vi "GUI_TRA_TREX.vi"() -> ()   [LabVIEW 2013]
uses:
  Device Drivers/TRAServer/HomingType_TypDef.ctl
  Device Drivers/TRAServer/StatusTRA_TypDef.ctl
  Device Drivers/shared/OnOffTypeDef.ctl
  <vilib>/Utility/file.llb/Write To Spreadsheet File (string).vi
  Device Drivers/TRAServer/TRAServer.lvclass
panel:
  in  "Multicolumn Listbox 2":refnum<vi>
  in  "Main Tap 2":refnum<vi>
  out "all pos array":refnum<vi>[][](array[refnum])
  out "all status array":refnum<vi>[][](array[refnum])
  out "indecator ref array 2":refnum<vi>[](array[refnum])
  out "indecator ref array":refnum<vi>[](array[refnum])
  in  "time to wait (TCP) 2":i32=10
  in  "plot":bool=TRUE
  out "ratio(h)":bool
  out "fixsize":bool
  out "error (h)":bool
  out "Device Name (h)":string="StagingTRA1"
  in  "Main Tap":T1(tab)
  in  "stepSize":dbl=0.01
  in  "Status":T2=enum."DISABLE" caption="Status Y"
  in  "Up":bool
  in  "Down":bool
  in  "Right":bool
  in  "Left":bool
  in  "Status":T2=enum."DISABLE" caption="Status X"
  in  "Position":dbl=2.54999 caption="X"
  in  "Position":dbl=3.05 caption="Y"
  in  "Mirror":enum16{"M20", "Switch", "M22", "M23"}(ring)
  in  "device status":string
  in  "Home 3":bool=TRUE
  in  "Home 2":bool=TRUE
  out "Status.Axis 6":T2=enum."DISABLE" caption="Status X"
  out "Status.Axis 5":T2=enum."DISABLE" caption="Status X"
  out "Status.Axis 4":T2=enum."DISABLE" caption="Status X"
  out "Status.Axis 3":T2=enum."DISABLE" caption="Status X"
  out "Status.Axis 2":T2=enum."DISABLE" caption="Status X"
  out "Status.Axis 1":T2=enum."DISABLE" caption="Status X"
  out "Status.Axis 1":T2=enum."DISABLE" caption="Status X"
  out "Status.Axis 2":T2=enum."DISABLE" caption="Status X"
  out "Status.Axis 3":T2=enum."DISABLE" caption="Status X"
  out "Status.Axis 4":T2=enum."DISABLE" caption="Status X"
  out "Status.Axis 5":T2=enum."DISABLE" caption="Status X"
  out "Status.Axis 6":T2=enum."DISABLE" caption="Status X"
  out "Status.Axis 7":T2=enum."DISABLE" caption="Status X"
  out "Status.Axis 8":T2=enum."DISABLE" caption="Status X"
  out "Status.Axis 9":T2=enum."DISABLE" caption="Status X"
  out "Status.Axis 10":T2=enum."DISABLE" caption="Status X"
  out "Status.Axis 11":T2=enum."DISABLE" caption="Status X"
  out "Status.Axis 12":T2=enum."DISABLE" caption="Status X"
  in  "Home 1":bool=TRUE
  in  "Path":path
  in  "Save":bool
  in  "Multicolumn Listbox":i32(listbox)
  in  "Position.Axis 1":dbl=3.05 caption="X"
  in  "Position.Axis 2":dbl=3.05 caption="Y"
  in  "Position.Axis 4":dbl=3.05 caption="X"
  in  "Position.Axis 3":dbl=3.05 caption="Y"
  in  "Position.Axis 6":dbl=3.05 caption="X"
  in  "Position.Axis 5":dbl=3.05 caption="Y"
  in  "Position.Axis 18":dbl=3.05 caption="X"
  in  "Position.Axis 17":dbl=3.05 caption="Y"
  in  "Position.Axis 16":dbl=3.05 caption="X"
  in  "Position.Axis 15":dbl=3.05 caption="Y"
  in  "Position.Axis 14":dbl=3.05 caption="X"
  in  "Position.Axis 13":dbl=3.05 caption="Y"
  in  "Position.Axis 12":dbl=3.05 caption="X"
  in  "Position.Axis 11":dbl=3.05 caption="Y"
  in  "Position.Axis 10":dbl=3.05 caption="X"
  in  "Position.Axis 9":dbl=3.05 caption="Y"
  in  "Position.Axis 8":dbl=3.05 caption="Y"
  in  "Position.Axis 7":dbl=3.05 caption="X"
  in  "Boolean":bool
  out "local Port":u16=65435
  in  "timeout ms (slow resp)":i32=500
  in  "reset":bool
  out "image con closed":bool
  out "image \nconnection":bool
  out "image con closed 2":bool
  out "All Devices (h)":string[](array[string])=["StagingTRA1"]
  out "Remote Host":string="192.168.11.97"
  out "port or service name":u16=65434
  out "port or service name out":u16=65400
  in  "time to wait (TCP)":i32=10
  out "error out":errorcluster
  out "connections (hidden)":variant[](array[variant])=[variant(refnum<k16> refnum), variant(refnum<k16> refnum)]
  in  "time to wait (main loop)":i32=10
  out "Data String":string="Position.Axis 1,2.549990000000\r\nStatus.Axis 1,DISABLE\r\nHomingType.Axis 1,EoR- switch only\r\nDisable.Axis 1,on\r\nDisable.Axis 2,on\r\nStatus.Axis 2,DISABLE\r\nPosition.Axis 2,3.050000000000\r\n"
  in  "Local Saving Path":path
  out "Nr.":i32
  out "error (h) 2":bool
  in  "shotnumber":i32
  out "String":string="wait>>Status.Axis 1,Status.Axis 2,Status.Axis 3,Status.Axis 4,Status.Axis 5,Status.Axis 6,Position.Axis 1,Position.Axis 2,Position.Axis 3,Position.Axis 4,Position.Axis 5,Position.Axis 6,Disable.Axis 1,Disable.Axis 2,Disable.Axis 3,Disable.Axis 4,Disable.Axis 5,Disable.Axis 6,HomingType.Axis 1,HomingType.Axis 2,HomingType.Axis 3,HomingType.Axis 4,HomingType.Axis 5,HomingType.Axis 6,Home.Axis 1,Home.Axis 2,Home.Axis 3,Home.Axis 4,Home.Axis 5,Home.Axis 6,Limits.pos.Axis 1,Limits.pos.Axis 2,Limits.pos.Axis 3,Limits.pos.Axis 4,Limits.pos.Axis 5,Limits.pos.Axis 6,Limits.neg.Axis 1,Limits.neg.Axis 2,Limits.neg.Axis 3,Limits.neg.Axis 4,Limits.neg.Axis 5,Limits.neg.Axis 6,TargetPos.Axis 1,TargetPos.Axis 2,TargetPos.Axis 3,TargetPos.Axis 4,TargetPos.Axis 5,TargetPos.Axis 6,backlash.Axis 1,backlash.Axis 2,backlash.Axis 3,backlash.Axis 4,backlash.Axis 5,backlash.Axis 6"
  in  "Limits.pos":dbl=2.54999
  in  "Home":T3=enum."on"
  in  "Disable":T3=enum."on"
  in  "HomingType":T4=enum."EoR- switch only"
  in  "Disable":T3=enum."on"
  in  "HomingType":T4=enum."EoR- switch only"
  in  "Home":T3=enum."on"
  in  "Limits.pos":dbl=2.54999
  in  "Limits.neg":dbl=2.54999
  in  "Limits.neg":dbl=2.54999
  in  "Mirror 2":enum16{"M20", "Switch", "M22", "M23"}(ring)
  in  "backlash 2":dbl
  in  "backlash":dbl
  out "error message":string
  out "Data Connection out":bool=TRUE
  # "Position"
  # "Chassi 1"
  # "Chassi 2"
  # "Chassi 3"
  # "X"
  # "Y"
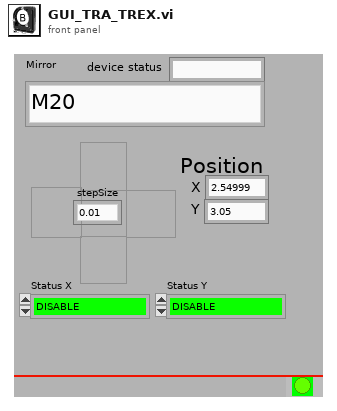
[diagram p1: front panel]
types:
  T1 = enum32{"Main", "Status", "Position", "Position 2", "Temp", "Network", "Internal", "MotorSettings"}
  T2 = typedef "TRAServer.lvclass/StatusTRA_TypDef.ctl" = enum16{"NOT REFERENCED", "CONFIGURATION", "HOMING", "MOVING", "READY", "DISABLE", "JOGGING"}
  T3 = typedef "OnOffTypeDef.ctl" = enum16{"off", "on"}
  T4 = typedef "TRAServer.lvclass/HomingType_TypDef.ctl" = enum16{"MZ switch and encoder Index", "current position as HOME", "MZ switch only", "EoR- switch and encoder Index", "EoR- switch only"}
  T5 = cluster{"Chassi Nr":i32, "X":string, "Y":string, "name":string}[]
  T6 = cluster{"Chassi Nr":i32, "X":string, "Y":string, "name":string}
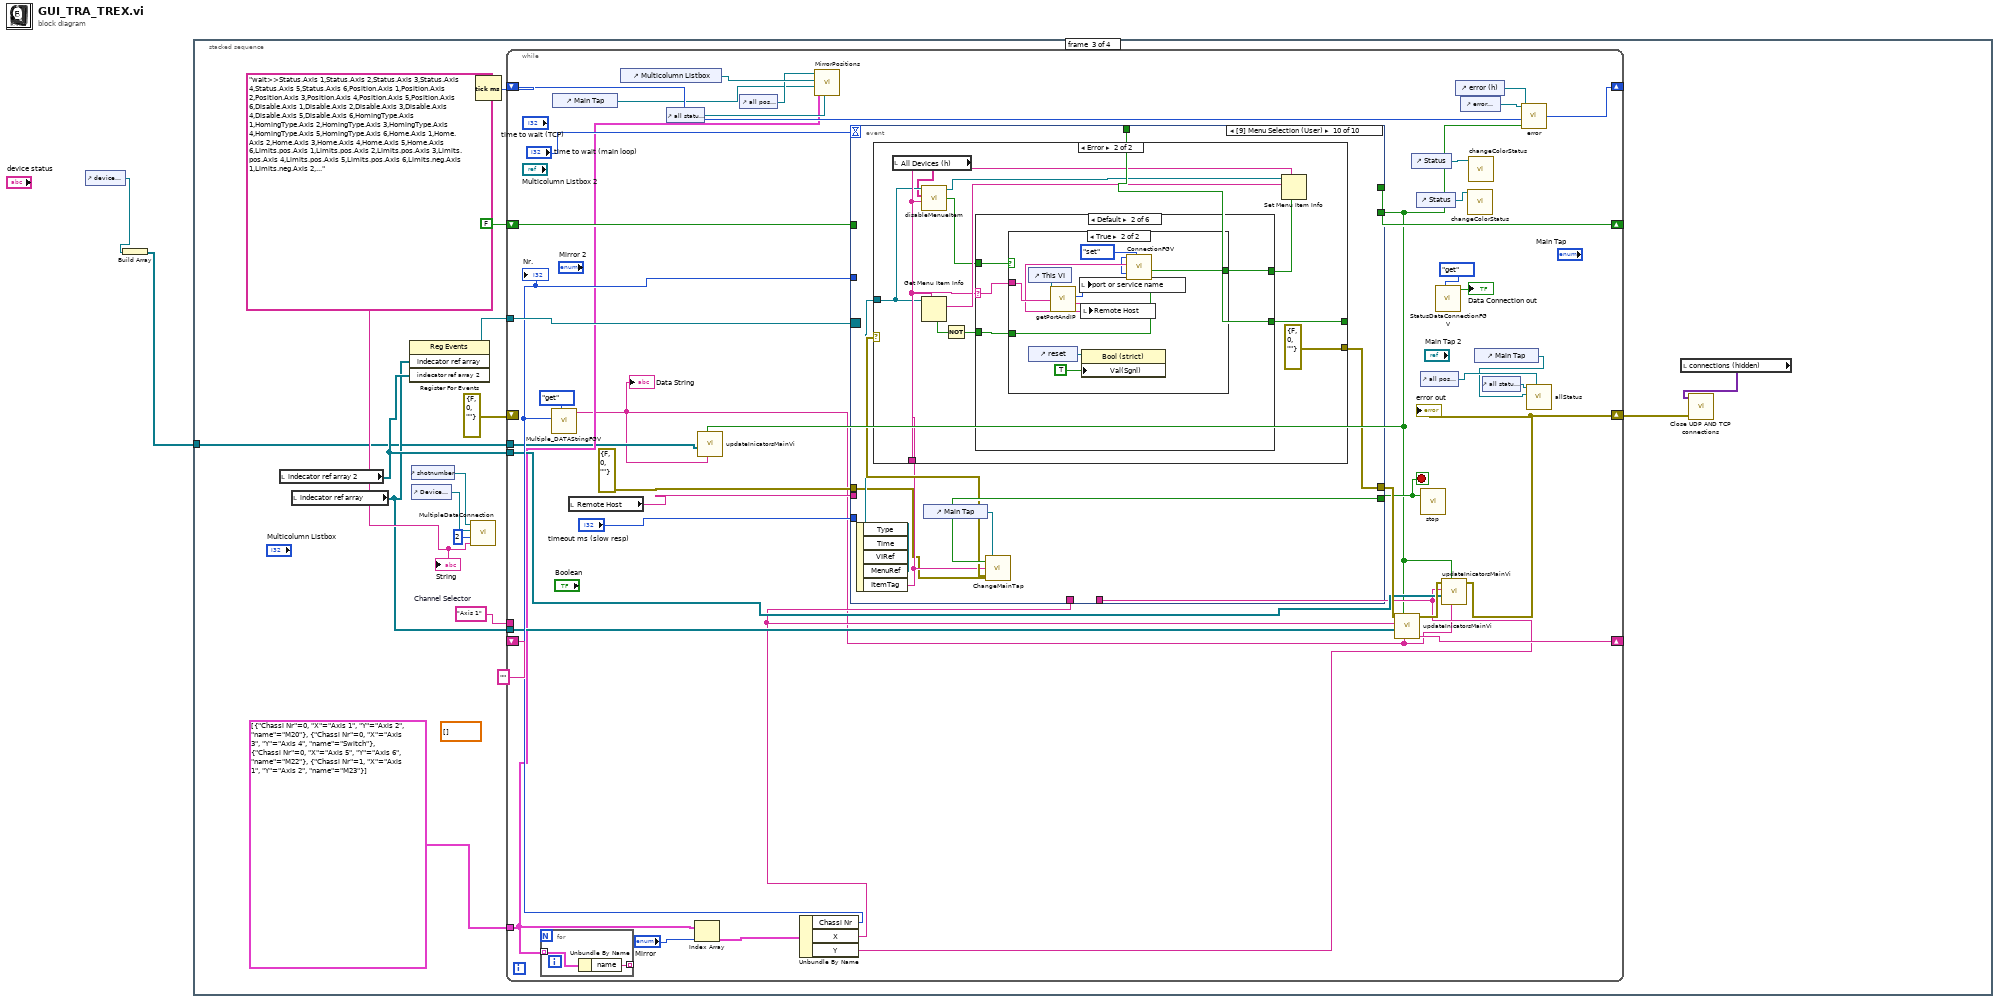
[diagram p0: block diagram]
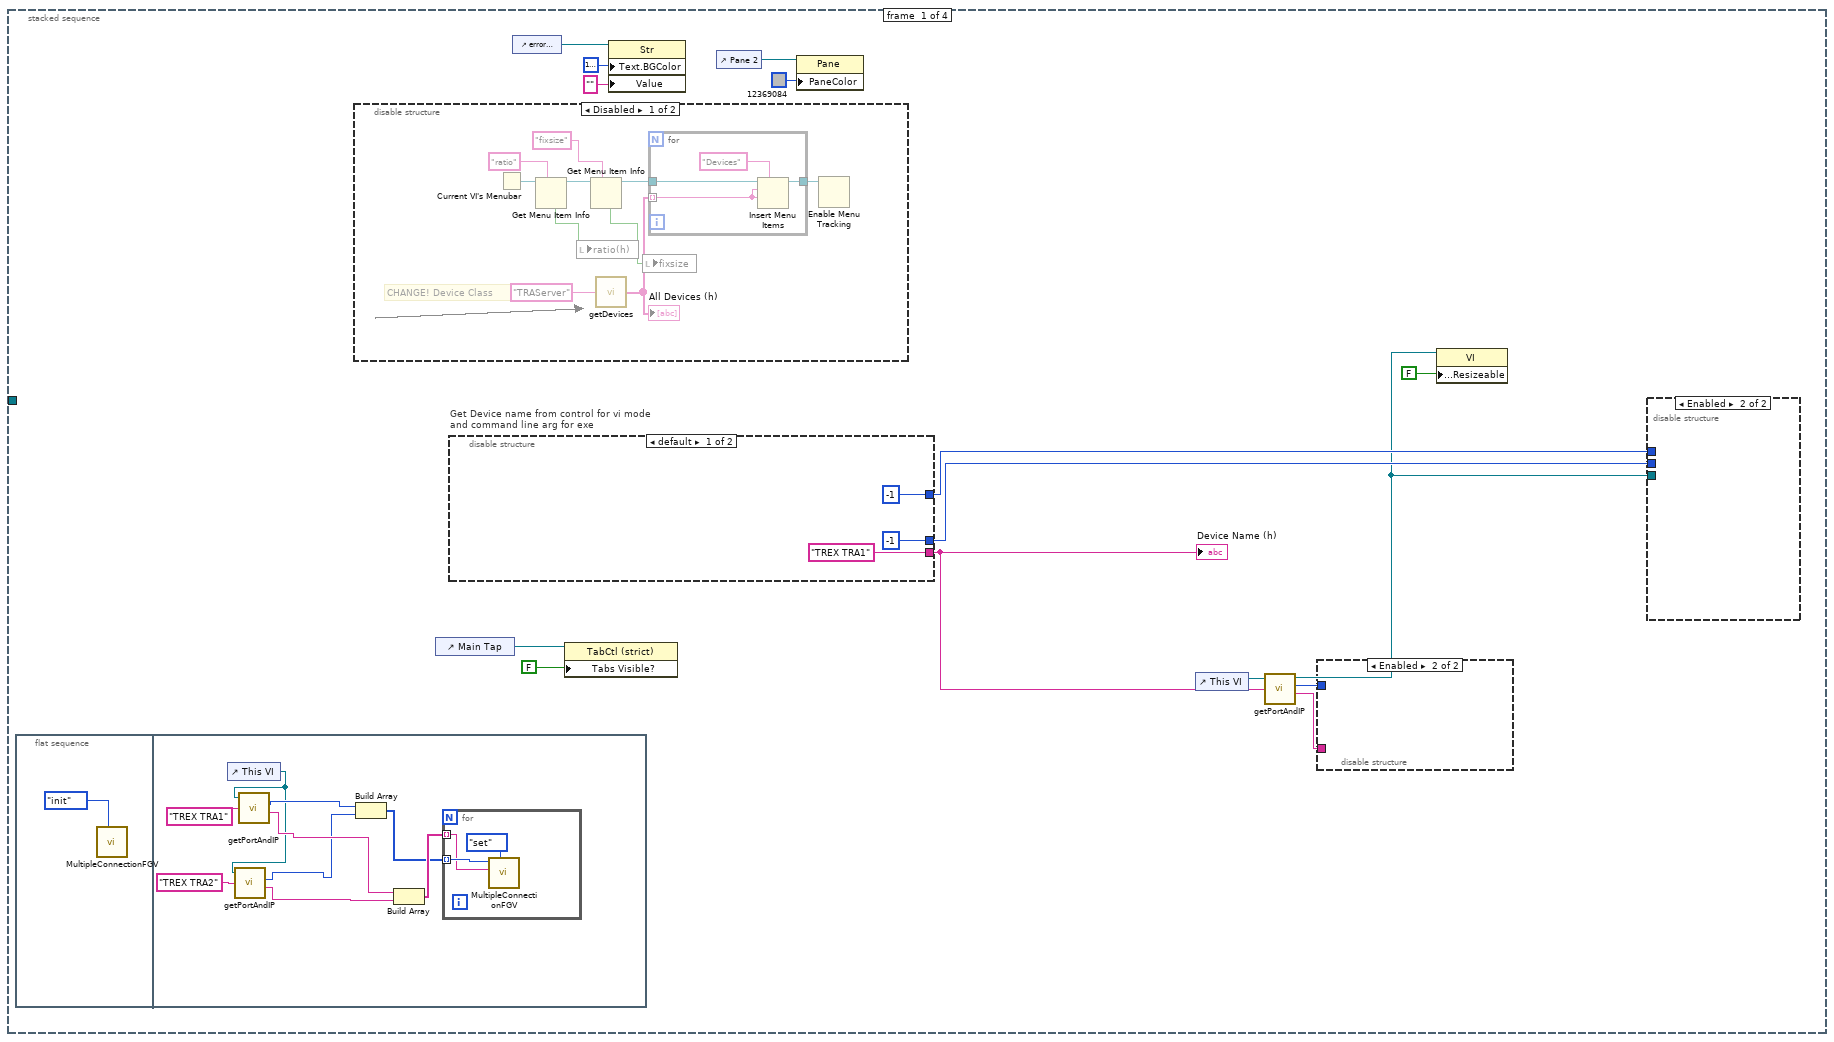
[diagram p2: hidden frame]
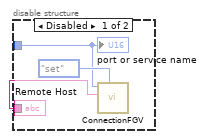
[diagram p4: hidden frame]
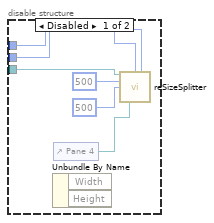
[diagram p5: hidden frame]
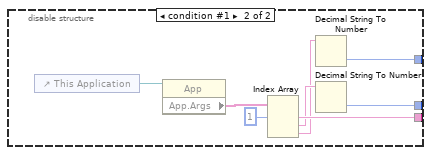
[diagram p6: hidden frame]
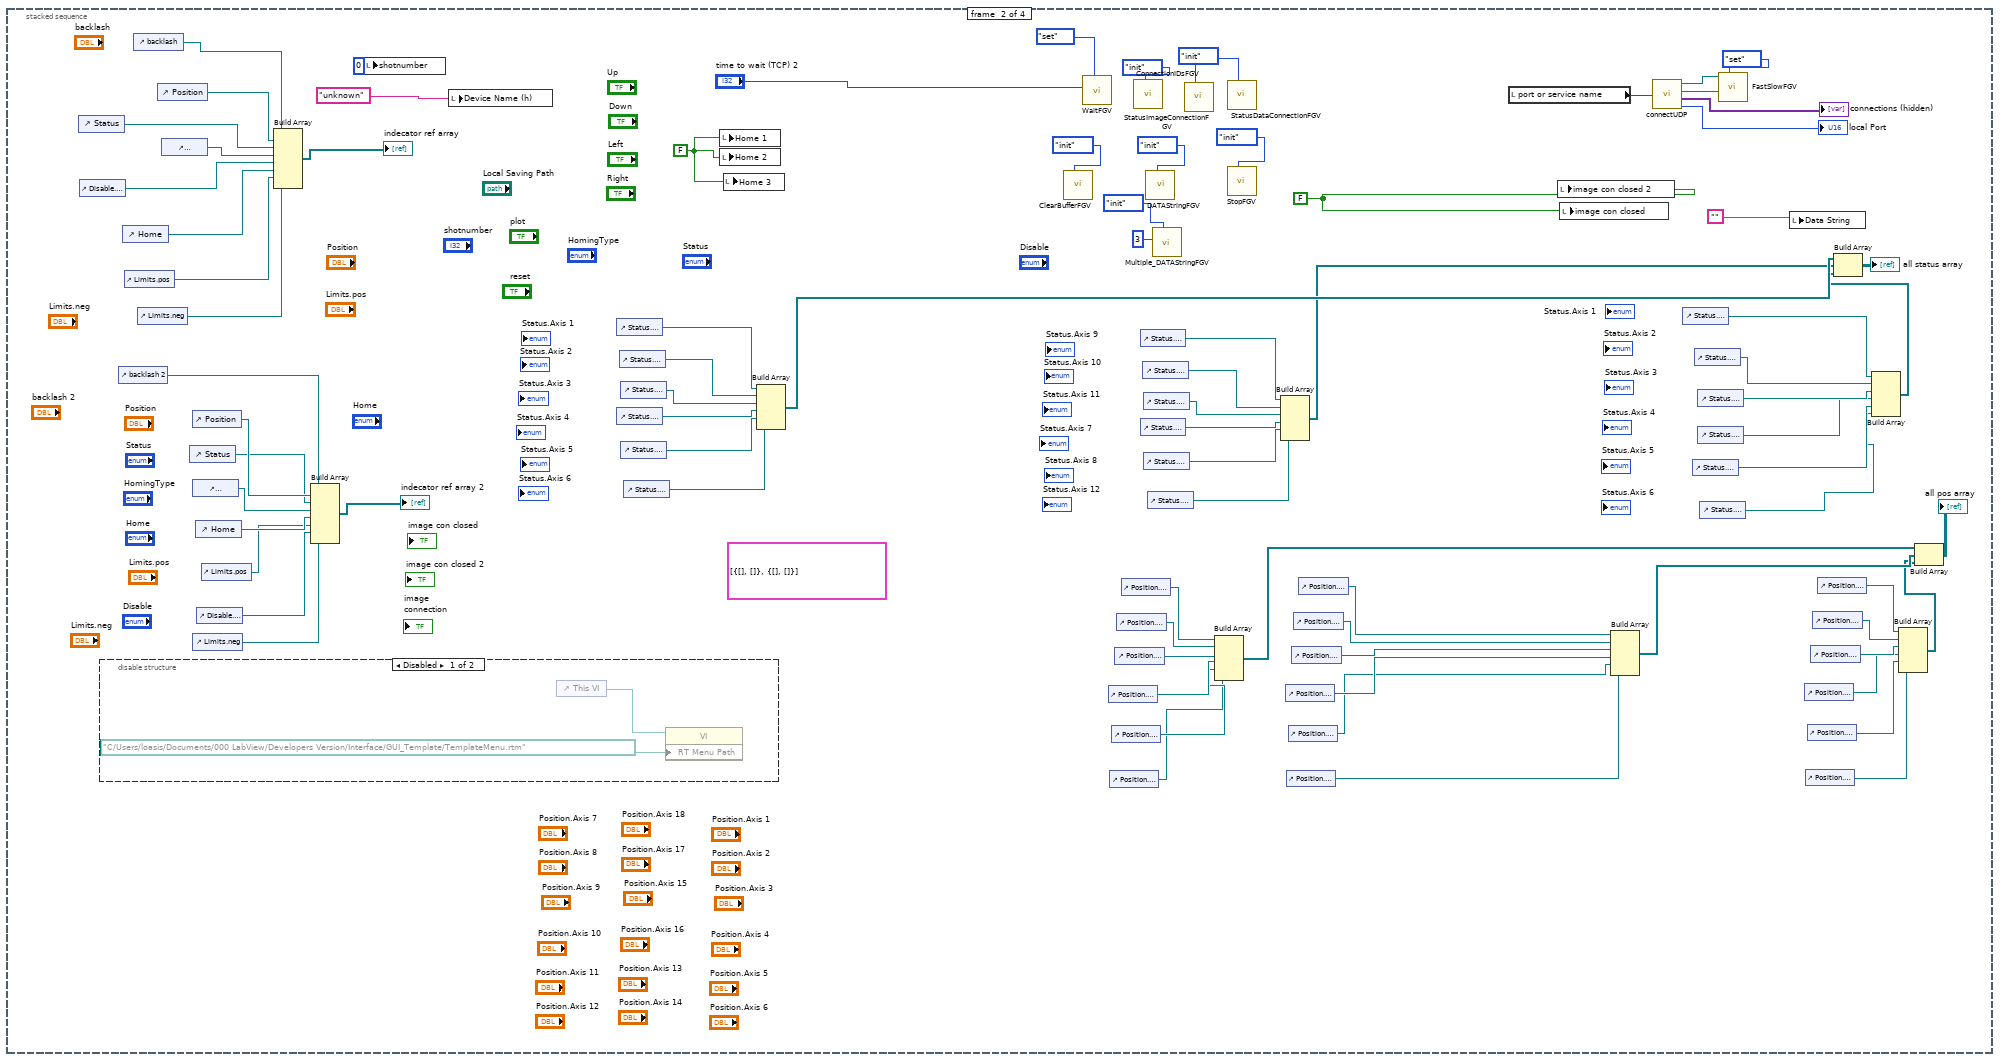
[diagram p7: hidden frame]
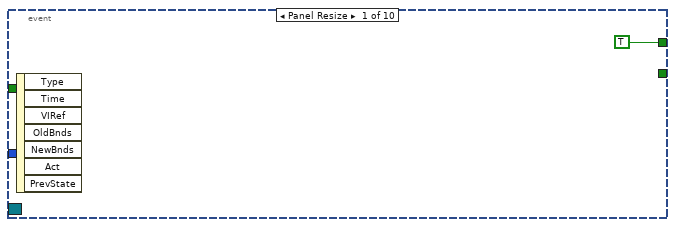
[diagram p9: hidden frame]
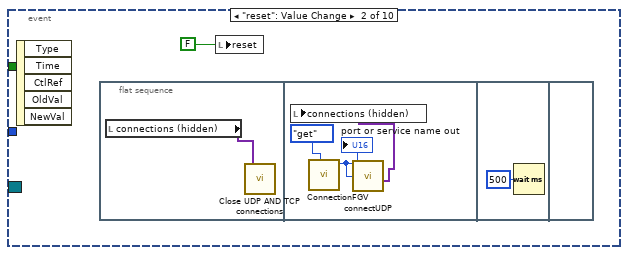
[diagram p10: hidden frame]
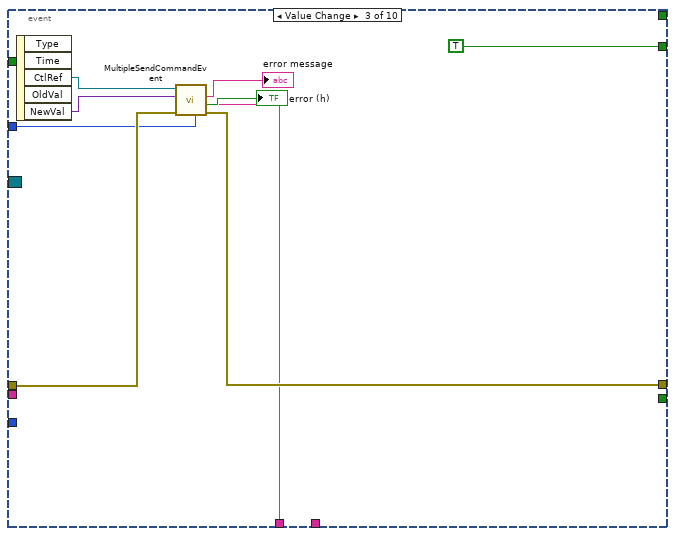
[diagram p11: hidden frame]
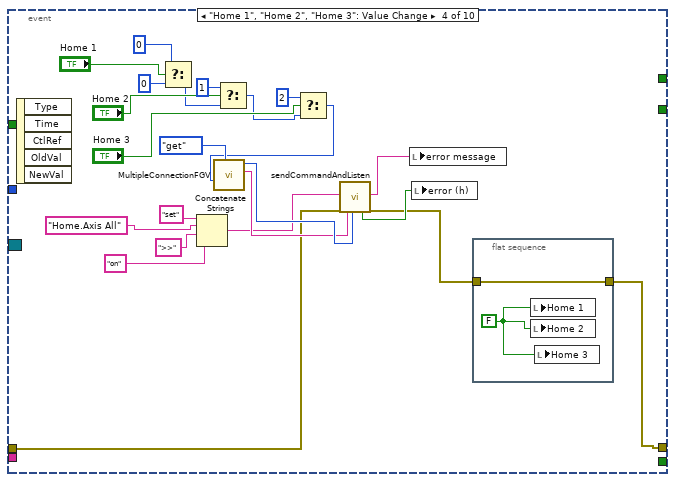
[diagram p12: hidden frame]
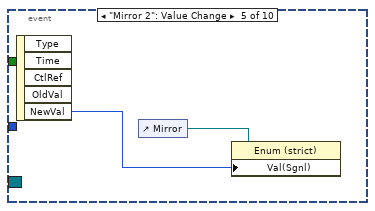
[diagram p13: hidden frame]
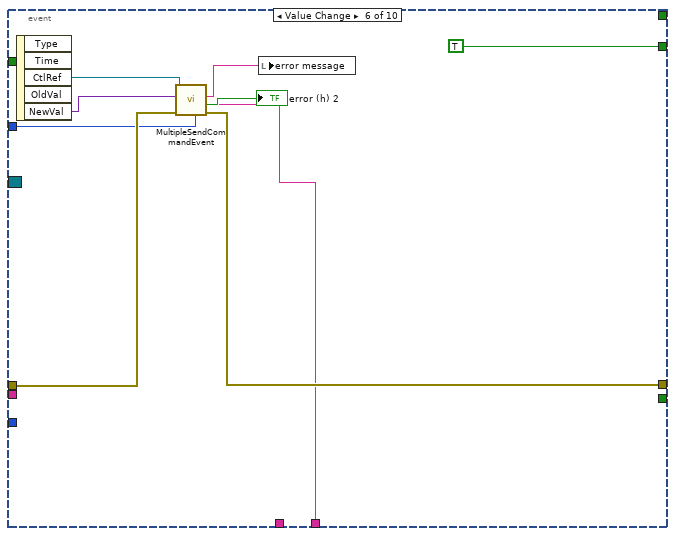
[diagram p14: hidden frame]
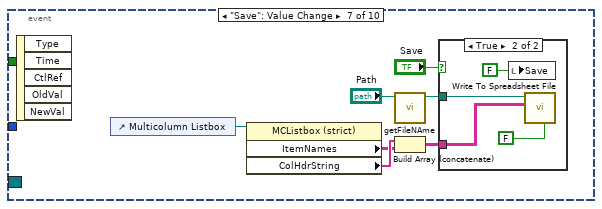
[diagram p15: hidden frame]
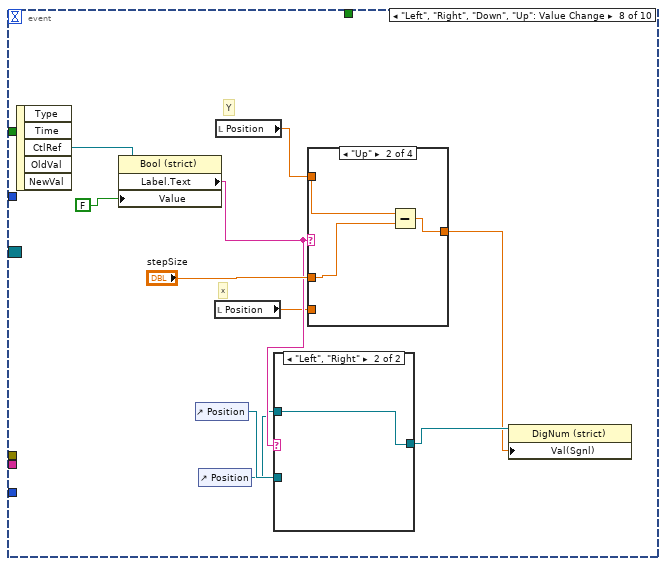
[diagram p17: hidden frame]
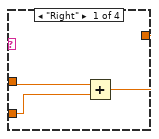
[diagram p19: hidden frame]
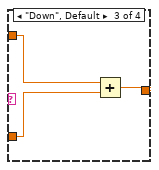
[diagram p20: hidden frame]
diagram:
  n1 = control-ref of="device status"() -> (w2:refnum<vi>)
  n2 = Build Array(w2) -> (w1:refnum<vi>[])
  n3 = stacked-sequence {
    tunnel: w1 -> [_ _ w149 _]
    frame #0 {
      n4 = flat-sequence {
        frame #0 {
          n5 = call "MultipleConnectionFGV.vi"("command"=enum16{"get", "set", "init"}."init") -> ()  [unwired: 9 in, 2 out]
        }
        frame #1 {
          n6 = control-ref of="This VI"() -> (w35:refnum<vi>)
          n7 = call "getPortAndIP.vi"("Device Name"="TREX TRA2", "This Vi"=w35) -> ("Remote Host"=w34:string, "port or service name"=w33:u16)  [unwired: 2 in, 3 out]
          n8 = call "getPortAndIP.vi"("Device Name"="TREX TRA1", "This Vi"=w35) -> ("Remote Host"=w38:string, "port or service name"=w37:u16)  [unwired: 2 in, 3 out]
          n9 = Build Array(w37, w33) -> (w40:u16[])
          n10 = Build Array(w38, w34) -> (w41:string[])
          n11 = for {
            tunnel: w40 -> [w43] mode=indexing
            tunnel: w41 -> [w42] mode=indexing
            n12 = call "MultipleConnectionFGV.vi"("command"=enum16{"get", "set", "init"}."set", "Remote Host in"=w42, "port or service name in"=w43) -> ()  [unwired: 7 in, 2 out]
          }
        }
      }
      n13 = disable-structure shown="Disabled" {
        frame Disabled {
          # "CHANGE! Device Class"
          n14 = Current VI's Menubar() -> (w26:refnum<k9>)
          n15 = Get Menu Item Info(7:"ratio" ("item tag"), 11:w26) -> (3:w24:refnum<k9>, 4:w25:bool)  [unwired: 1 in, 5 out]
          n16 = local write "ratio(h)"(w25) -> ()
          n17 = Get Menu Item Info(7:"fixsize" ("item tag"), 11:w24) -> (3:w21:refnum<k9>, 4:w22:bool)  [unwired: 1 in, 5 out]
          n18 = call "getDevices.vi"("Device Class"="TRAServer") -> ("All Devices"=w19:string[])
          "All Devices (h)" <- w19
          n19 = local write "fixsize"(w22) -> ()
          n20 = for {
            tunnel: w21 -> [w31]
            tunnel: [w30] -> w20
            tunnel: w19 -> [w28] mode=indexing
            n21 = Insert Menu Items(5:"Devices" ("menu tag"), 7:w28, 8:w28, 9:w31) -> (3:w30:refnum<k9>)  [unwired: 2 in, 2 out]
          }
          n22 = Enable Menu Tracking(4:w20) -> ()  [unwired: 2 in, 2 out]
        }
        frame Enabled {
        }
      }
      n23 = control-ref of="Main Tap"() -> (w17:refnum<vi>)
      n24 = disable-structure "Get Device name from control for vi mode\nand command line arg for exe" shown="default" {
        disable-tunnel: ["TREX TRA1" ("Device Name for vi mode") w61] -> w13
        disable-tunnel: [i16 -1 ("left") w58] -> w15
        disable-tunnel: [i16 -1 ("left") w57] -> w14
        frame condition #0 (active) {
        }
        frame condition #1 {
          n25 = control-ref of="This Application"() -> (w64:refnum<vi>)
          n26 = property class="App"(reference=w64) -> ("App.Args"=w63:string[])  [unwired: 1 in, 2 out]
          n27 = Index Array(array=w63, index #1=1 ("index")) -> (element #1=w61:string, element #2=w60:string, element #3=w59:string)  [unwired: 2 in]
          n28 = Decimal String To Number(string=w59) -> (number=w57:i32)  [unwired: 2 in, 1 out]
          n29 = Decimal String To Number(string=w60) -> (number=w58:i32)  [unwired: 2 in, 1 out]
        }
      }
      "Device Name (h)" <- w13
      n30 = control-ref of="error message"() -> (w6:refnum<vi>)
      n31 = property class="TabCtl (strict)"(reference=w17, "Tabs Visible?"=FALSE) -> ()  [unwired: 1 in, 2 out]
      n32 = property class="Str"(reference=w6, "Text.BGColor"=u32 16777238, "Value"="") -> ()  [unwired: 1 in, 2 out]
      n33 = control-ref of="Pane 2"() -> (w4:refnum<vi>)
      n34 = property class="Pane"(reference=w4, "PaneColor"=u32 12369084) -> ()  [unwired: 1 in, 2 out]
      n35 = control-ref of="This VI"() -> (w12:refnum<vi>)
      n36 = call "getPortAndIP.vi"("Device Name"=w13, "This Vi"=w12) -> ("Remote Host"=w9:string, "port or service name"=w8:u16, "reference out"=w10:refnum<vi>)  [unwired: 2 in, 2 out]
      n37 = disable-structure shown="Enabled" {
        disable-tunnel: w9 -> [w46 _]
        disable-tunnel: w8 -> [w45 _]
        frame Disabled {
          n38 = call "ConnectionFGV.vi"("command"=enum16{"get", "set", "init"}."set", "Remote Host in"=w46, "port or service name in"=w45) -> ()  [unwired: 7 in, 2 out]
          "port or service name" <- w45
          "Remote Host" <- w46
        }
        frame Enabled {
        }
      }
      n39 = property class="VI"(reference=w10, "Front Panel.Resizeable"=FALSE ("Front Panel Window:Resizable")) -> ()  [unwired: 1 in, 2 out]
      n40 = disable-structure shown="Enabled" {
        disable-tunnel: w15 -> [w53 _]
        disable-tunnel: w14 -> [w52 _]
        disable-tunnel: w10 -> [w50 _]
        frame Disabled {
          n41 = Unbundle By Name() -> ()  [unwired: 1 in, 2 out]
          n42 = control-ref of="Pane 4"() -> (w51:refnum<vi>)
          n43 = call "reSizeSplitter.vi"("this vi"=w50, "left"=w53, "top"=w52, "Width"=u32 500, "Height"=u32 500, "pane2"=w51) -> ()  [unwired: 9 in, 1 out]
        }
        frame Enabled {
        }
      }
    }
    frame #1 {
      (unwired) cluster{dbl[], dbl[]}[] [{[], []}, {[], []}] ("appended array 4")
      w89 = FALSE
      w138 = enum16{"get", "set", "init"}."init" ("Command")
      w144 = FALSE ("new Device Data")
      n44 = control-ref of="Status"() -> (w127:refnum<vi>)
      n45 = control-ref of="Disable.Axis 1"() -> (w125:refnum<vi>)
      n46 = disable-structure shown="Disabled" {
        frame Disabled {
          n47 = control-ref of="This VI"() -> (w148:refnum<vi>)
          n48 = property class="VI"(reference=w148, "RT Menu Path"=path "C:/Users/loasis/Documents/000 LabView/Developers Version/Interface/GUI_Template/TemplateMenu.rtm" ("Run-Time Menu Path")) -> ()  [unwired: 1 in, 2 out]
        }
        frame Enabled {
        }
      }
      n49 = control-ref of="backlash 2"() -> (w66:refnum<vi>)
      n50 = control-ref of="Home"() -> (w124:refnum<vi>)
      n51 = control-ref of="Limits.pos"() -> (w123:refnum<vi>)
      n52 = control-ref of="backlash"() -> (w65:refnum<vi>)
      n53 = control-ref of="Limits.neg"() -> (w113:refnum<vi>)
      n54 = control-ref of="Position"() -> (w128:refnum<vi>)
      n55 = control-ref of="HomingType.Axis 1"() -> (w126:refnum<vi>)
      n56 = control-ref of="Status"() -> (w119:refnum<vi>)
      n57 = control-ref of="Position"() -> (w120:refnum<vi>)
      n58 = control-ref of="HomingType"() -> (w118:refnum<vi>)
      n59 = control-ref of="Limits.neg"() -> (w112:refnum<vi>)
      n60 = control-ref of="Home"() -> (w117:refnum<vi>)
      n61 = control-ref of="Disable.Axis"() -> (w115:refnum<vi>)
      n62 = control-ref of="Limits.pos"() -> (w116:refnum<vi>)
      n63 = Build Array(w65, w128, w127, w126, w125, w124, w123, w113) -> (→"indecator ref array":refnum<vi>[])
      n64 = Build Array(w66, w120, w119, w118, w117, w116, w115, w112) -> (→"indecator ref array 2":refnum<vi>[])
      n65 = local write "shotnumber"(0 ("shotnumber")) -> ()
      n66 = local write "Device Name (h)"("unknown" ("Device Name")) -> ()
      n67 = control-ref of="Status.Axis 1"() -> (w94:refnum<vi>)
      n68 = control-ref of="Status.Axis 4"() -> (w97:refnum<vi>)
      n69 = control-ref of="Status.Axis 2"() -> (w95:refnum<vi>)
      n70 = control-ref of="Status.Axis 3"() -> (w96:refnum<vi>)
      n71 = control-ref of="Status.Axis 5"() -> (w98:refnum<vi>)
      n72 = control-ref of="Status.Axis 6"() -> (w99:refnum<vi>)
      n73 = local write "Home 1"(w89) -> ()
      n74 = local write "Home 2"(w89) -> ()
      n75 = local write "Home 3"(w89) -> ()
      n76 = Build Array(w94, w95, w96, w97, w98, w99) -> (w93:refnum<vi>[])
      n77 = call "ClearBufferFGV.vi"("Command"=enum16{"set", "get", "init"}."init") -> ()  [unwired: 10 in, 1 out]
      n78 = call "WaitFGV.vi"("Command"=enum16{"get", "set", "init"}."set", "milliseconds to wait"="time to wait (TCP) 2") -> ()  [unwired: 9 in, 1 out]
      n79 = control-ref of="Position.Axis 10"() -> (w85:refnum<vi>)
      n80 = control-ref of="Position.Axis 12"() -> (w83:refnum<vi>)
      n81 = control-ref of="Position.Axis 11"() -> (w84:refnum<vi>)
      n82 = control-ref of="Position.Axis 9"() -> (w86:refnum<vi>)
      n83 = control-ref of="Position.Axis 8"() -> (w87:refnum<vi>)
      n84 = control-ref of="Position.Axis 7"() -> (w88:refnum<vi>)
      n85 = call "ConnectionIDsFGV.vi"("Command"=enum16{"add", "get", "init"}."init") -> ()  [unwired: 10 in, 1 out]
      n86 = control-ref of="Status.Axis 9"() -> (w105:refnum<vi>)
      n87 = control-ref of="Status.Axis 7"() -> (w102:refnum<vi>)
      n88 = control-ref of="Status.Axis 10"() -> (w104:refnum<vi>)
      n89 = control-ref of="Status.Axis 11"() -> (w103:refnum<vi>)
      n90 = control-ref of="Status.Axis 8"() -> (w101:refnum<vi>)
      n91 = call "DATAStringFGV.vi"("Command"=enum16{"get", "set", "init"}."init") -> ()  [unwired: 9 in, 2 out]
      n92 = control-ref of="Status.Axis 12"() -> (w100:refnum<vi>)
      n93 = call "Multiple_DATAStringFGV.vi"("Command"=enum16{"get", "set", "init"}."init", "Nr."=3) -> ()  [unwired: 9 in, 1 out]
      n94 = call "StatusImageConnectionFGV.vi"("Command"=w138) -> ()  [unwired: 10 in, 1 out]
      n95 = Build Array(w88, w87, w86, w85, w84, w83) -> (w70:refnum<vi>[])
      n96 = call "StatusDataConnectionFGV.vi"("Command"=w138) -> ()  [unwired: 10 in, 1 out]
      n97 = call "StopFGV.vi"("Command"=enum16{"set", "get", "init"}."init") -> ()  [unwired: 9 in, 2 out]
      n98 = Build Array(w105, w104, w103, w102, w101, w100) -> (w92:refnum<vi>[])
      n99 = control-ref of="Position.Axis 16"() -> (w79:refnum<vi>)
      n100 = control-ref of="Position.Axis 14"() -> (w77:refnum<vi>)
      n101 = control-ref of="Position.Axis 13"() -> (w78:refnum<vi>)
      n102 = control-ref of="Position.Axis 15"() -> (w80:refnum<vi>)
      n103 = control-ref of="Position.Axis 17"() -> (w81:refnum<vi>)
      n104 = control-ref of="Position.Axis 18"() -> (w82:refnum<vi>)
      n105 = local read "port or service name"() -> (w134:u16)
      n106 = local write "image con closed 2"(w144) -> ()
      n107 = local write "image con closed"(w144) -> ()
      n108 = Build Array(w82, w81, w80, w79, w78, w77) -> (w69:refnum<vi>[])
      n109 = call "connectUDP.vi"("port or service name NOT USED"=w134) -> ("fast ID (h)"=w133:refnum<k16>, "slow ID (h)"=w132:refnum<k16>, "connections (hidden)"=→"connections (hidden)":variant[], "local Port"=→"local Port":u16)
      n110 = control-ref of="Status.Axis 1"() -> (w111:refnum<vi>)
      n111 = control-ref of="Status.Axis 5"() -> (w107:refnum<vi>)
      n112 = control-ref of="Status.Axis 2"() -> (w110:refnum<vi>)
      n113 = control-ref of="Status.Axis 3"() -> (w109:refnum<vi>)
      n114 = control-ref of="Status.Axis 4"() -> (w108:refnum<vi>)
      n115 = control-ref of="Status.Axis 6"() -> (w106:refnum<vi>)
      n116 = call "FastSlowFGV.vi"("Command"=enum16{"get", "set", "init"}."set", "slow ID"=w132, "fast ID"=w133) -> ()  [unwired: 7 in, 2 out]
      n117 = local write "Data String"("") -> ()
      n118 = control-ref of="Position.Axis 4"() -> (w73:refnum<vi>)
      n119 = control-ref of="Position.Axis 6"() -> (w71:refnum<vi>)
      n120 = control-ref of="Position.Axis 5"() -> (w72:refnum<vi>)
      n121 = control-ref of="Position.Axis 3"() -> (w74:refnum<vi>)
      n122 = control-ref of="Position.Axis 2"() -> (w75:refnum<vi>)
      n123 = control-ref of="Position.Axis 1"() -> (w76:refnum<vi>)
      n124 = Build Array(w111, w110, w109, w108, w107, w106) -> (w91:refnum<vi>[])
      n125 = Build Array(w93, w92, w91) -> (→"all status array":refnum<vi>[][])
      n126 = Build Array(w76, w75, w74, w73, w72, w71) -> (w68:refnum<vi>[])
      n127 = Build Array(w70, w69, w68) -> (→"all pos array":refnum<vi>[][])
    }
    frame #2 {
      w153 = "wait>>Status.Axis 1,Status.Axis 2,Status.Axis 3,Status.Axis 4,Status.Axis 5,Status.Axis 6,Position.Axis 1,Position.Axis 2,Position.Axis 3,Position.Axis 4,Position.Axis 5,Position.Axis 6,Disable.Axis 1,Disable.Axis 2,Disable.Axis 3,Disable.Axis 4,Disable.Axis 5,Disable.Axis 6,HomingType.Axis 1,HomingType.Axis 2,HomingType.Axis 3,HomingType.Axis 4,HomingType.Axis 5,HomingType.Axis 6,Home.Axis 1,Home.Axis 2,Home.Axis 3,Home.Axis 4,Home.Axis 5,Home.Axis 6,Limits.pos.Axis 1,Limits.pos.Axis 2,Limits.pos.Axis 3,Limits.pos.Axis 4,Limits.pos.Axis 5,Limits.pos.Axis 6,Limits.neg.Axis 1,Limits.neg.Axis 2,Limits.neg.Axis 3,Limits.neg.Axis 4,Limits.neg.Axis 5,Limits.neg.Axis 6,TargetPos.Axis 1,TargetPos.Axis 2,TargetPos.Axis 3,TargetPos.Axis 4,TargetPos.Axis 5,TargetPos.Axis 6,backlash.Axis 1,backlash.Axis 2,backlash.Axis 3,backlash.Axis 4,backlash.Axis 5,backlash.Axis 6,device status" ("String")
      (unwired) dbl[] []
      w155 = "Axis 1"  # Channel Selector
      n128 = local read "indecator ref array 2"() -> (w152:refnum<vi>[])
      n129 = local read "indecator ref array"() -> (w151:refnum<vi>[])
      n130 = register-events(w151, w152) -> (reference out=w156:refnum<event-registration>)  [unwired: 2 in, 1 out]
      n131 = control-ref of="shotnumber"() -> (w158:refnum<vi>)
      n132 = control-ref of="Device Name (h)"() -> (w157:refnum<vi>)
      n133 = call "MultipleDataConnection.vi"("Subscriber list 2"=w153, "Nr."=2, "Device Name (h)"=w157, "shotnumber"=w158) -> ()
      n134 = Tick Count (ms)() -> (millisecond timer value=w160:u32)
      n135 = while {
        shift-right: [w186] -> w163
        shift-left: errorcluster {"status"=FALSE, "code"=0, "source"=""} ("error out") -> [_]
        tunnel: w151 -> [w184]
        shift-right: [w198] -> _
        shift-left: FALSE -> [w199]
        shift-right: [w197] -> _
        shift-left: w160 -> [w196]
        shift-right: [w191] -> _
        shift-left: "" ("Data String") -> [_]
        tunnel: w156 -> [w193]
        tunnel: w155 -> [_]
        tunnel: w152 -> [w183]
        tunnel: T5 [{"Chassi Nr"=0, "X"="Axis 1", "Y"="Axis 2", "name"="M20"}, {"Chassi Nr"=0, "X"="Axis 3", "Y"="Axis 4", "name"="Switch"}, {"Chassi Nr"=0, "X"="Axis 5", "Y"="Axis 6", "name"="M22"}, {"Chassi Nr"=1, "X"="Axis 1", "Y"="Axis 2", "name"="M23"}] -> [w170]
        tunnel: w149 -> [w167]
        stop <- w194 stop-if-true
        n136 = for {
          tunnel: w170 -> [w205] mode=indexing
          tunnel: [w204] -> _ mode=indexing
          n137 = Unbundle By Name(w205) -> ("name"=w204:string)
        }
        n138 = control-ref of="Main Tap"() -> (w168:refnum<vi>)
        n139 = local read "Remote Host"() -> (w201:string)
        n140 = control-ref of="Multicolumn Listbox"() -> (w173:refnum<vi>)
        n141 = control-ref of="all status array"() -> (w171:refnum<vi>)
        n142 = Index Array(array=w170, index="Mirror") -> (element=w174:T6)
        n143 = control-ref of="all pos array"() -> (w172:refnum<vi>)
        n144 = Unbundle By Name(w174) -> ("Chassi Nr"=w185:i32, "X"=w182:string, "Y"=w181:string)
        "Nr." <- w185
        n145 = call "Multiple_DATAStringFGV.vi"("Command"=enum16{"get", "set", "init"}."get", "Nr."=w185) -> ("Data String out"=w165:string)  [unwired: 9 in]
        "Data String" <- w165
        n146 = call "MirrorPositions.vi"("all status array"=w171, "Array"=w170, "reference"=w168, "Multicolumn Listbox 2"=w173, "Array in"=w172) -> ()  [unwired: 7 in]
        n147 = event shown="[9] Menu Selection (User)" {
          selector: w193 -> [_ _ _ _ _ _ _ _ _ _]
          dyn-events: _ -> [_ _ _ _ _ _ _ _ _ _]
          timeout: "time to wait (main loop)" -> [_ _ _ _ _ _ _ _ _ _]
          tunnel: [_ _ w219 w222 _ w255 _ _ w294 w296] -> w200
          tunnel: w201 -> [_ _ _ _ _ _ _ _ _ _]
          tunnel: "timeout ms (slow resp)" -> [_ _ _ _ _ _ _ _ _ _]
          tunnel: errorcluster {"status"=FALSE, "code"=0, "source"=""} ("error out") -> [_ _ w216 w239 _ w253 _ _ w294 w297]
          tunnel: [_ _ TRUE _ _ TRUE _ _ _ _] -> w166
          tunnel: [_ _ _ _ _ _ _ _ _ w302] -> w194
          tunnel: [_ _ _ _ _ _ _ _ w293 w299] -> _
          tunnel: w199 -> [_ _ _ _ _ _ _ _ w293 _]
          tunnel: [TRUE _ _ _ _ _ _ _ _ _] -> w198
          tunnel: w185 -> [_ _ w214 _ _ w251 _ _ _ _]
          tunnel: w182 -> [_ _ w213 _ _ _ _ _ _ _]
          tunnel: w181 -> [_ _ _ _ _ w250 _ _ _ _]
          event Panel Resize {
            n148 = event-data() -> ()  [unwired: 1 in, 7 out]
          }
          event "reset": Value Change {
            n149 = event-data() -> ()  [unwired: 1 in, 5 out]
            n150 = flat-sequence {
              frame #0 {
                n151 = local read "connections (hidden)"() -> (w208:variant[])
                n152 = call "Close UDP AND TCP connections.vi"("appended array"=w208) -> ()  [unwired: 7 in]
              }
              frame #1 {
                n153 = call "ConnectionFGV.vi"("command"=enum16{"get", "set", "init"}."get") -> ("port or service name out"=w210:u16)  [unwired: 9 in, 1 out]
                "port or service name out" <- w210
                n154 = call "connectUDP.vi"("port or service name NOT USED"=w210) -> ("connections (hidden)"=w209:variant[])  [unwired: 3 out]
                n155 = local write "connections (hidden)"(w209) -> ()
              }
              frame #2 {
                n156 = Wait (ms)(milliseconds to wait=u32 500) -> ()  [unwired: 1 out]
              }
              frame #3 {
              }
            }
            n157 = local write "reset"(FALSE ("reset")) -> ()
          }
          event Value Change {
            n158 = event-data() -> ("CtlRef"=w221:refnum<vi>, "NewVal"=w220:variant)  [unwired: 1 in, 3 out]
            n159 = call "MultipleSendCommandEvent.vi"("Nr."=w214, "error out 2"=w216, "Channel Selector"=w213, "NewVal"=w220, "CtlRef"=w221) -> ("error out"=w219:errorcluster, "error (h)"=→"error (h)":bool, "error message"=→"error message":string)  [unwired: 3 in, 1 out]
          }
          event "Home 1", "Home 2", "Home 3": Value Change {
            n160 = event-data() -> ()  [unwired: 1 in, 5 out]
            n161 = Select(t=0 ("Nr."), s="Home 1", f=0) -> (s? t:f=w226:i32)
            n162 = Concatenate Strings("set", "Home.Axis All" ("string"), ">>" ("string"), "on" ("string")) -> (w241:string)
            n163 = Select(t=1 ("Nr."), s="Home 2", f=w226) -> (s? t:f=w227:i32)
            n164 = Select(t=2 ("Nr."), s="Home 3", f=w227) -> (s? t:f=w224:i32)
            n165 = call "MultipleConnectionFGV.vi"("command"=enum16{"get", "set", "init"}."get", "Nr."=w224) -> ("Remote Host out"=w243:string, "port or service name out"=w244:u16)  [unwired: 8 in]
            n166 = call "sendCommandAndListen.vi"("command in"=w241, "error in"=w239, "Remote Host"=w243, "port or service name"=w244) -> ("error"=w237:bool, "error message"=w238:string, "error out"=w223:errorcluster)  [unwired: 8 in, 5 out]
            n167 = local write "error message"(w238) -> ()
            n168 = local write "error (h)"(w237) -> ()
            n169 = flat-sequence {
              tunnel: w223 -> [w246]
              tunnel: [w246] -> w222
              frame #0 {
                w245 = FALSE
                n170 = local write "Home 1"(w245) -> ()
                n171 = local write "Home 2"(w245) -> ()
                n172 = local write "Home 3"(w245) -> ()
              }
            }
          }
          event "Mirror 2": Value Change {
            n173 = event-data() -> ("NewVal"=w247:enum16{"M20", "Switch", "M22", "M23"})  [unwired: 1 in, 4 out]
            n174 = control-ref of="Mirror"() -> (w248:refnum<vi>)
            n175 = property class="Enum (strict)"(reference=w248, "Val(Sgnl)"=w247) -> ()  [unwired: 1 in, 2 out]
          }
          event Value Change {
            n176 = event-data() -> ("CtlRef"=w257:refnum<vi>, "NewVal"=w256:variant)  [unwired: 1 in, 3 out]
            n177 = call "MultipleSendCommandEvent.vi"("Nr."=w251, "error out 2"=w253, "Channel Selector"=w250, "NewVal"=w256, "CtlRef"=w257) -> ("error out"=w255:errorcluster, "error (h)"=→"error (h) 2":bool, "error message"=w249:string)  [unwired: 3 in, 1 out]
            n178 = local write "error message"(w249) -> ()
          }
          event "Save": Value Change {
            n179 = event-data() -> ()  [unwired: 1 in, 5 out]
            n180 = control-ref of="Multicolumn Listbox"() -> (w264:refnum<vi>)
            n181 = property class="MCListbox (strict)"(reference=w264) -> ("ItemNames"=w262:string[][], "ColHdrString"=w263:string[])  [unwired: 1 in, 2 out]
            n182 = call "getFileNAme.vi"("Path"="Path") -> ("appended path"=w258:path)  [unwired: 9 in, 1 out]
            n183 = Build Array (concatenate)(w263, w262) -> (w260:string[][])
            n184 = case shown="True" "Save" {
              tunnel: w258 -> [_ w267]
              tunnel: w260 -> [_ w266]
              frame False {
              }
              frame True {
                n185 = local write "Save"(FALSE ("Save")) -> ()
                n186 = call-poly <vilib>:"Write To Spreadsheet File.vi"("transpose? (no:F)"=FALSE, "2D data"=w266, "file path (dialog if empty)"=w267) -> ()  [unwired: 5 in, 1 out]
              }
            }
          }
          event "Left", "Right", "Down", "Up": Value Change {
            # "Y"
            # "x"
            n187 = event-data() -> ("CtlRef"=w278:refnum<vi>)  [unwired: 1 in, 4 out]
            n188 = property class="Bool (strict)"(reference=w278, "Value"=FALSE) -> ("Label.Text"=w275:string)  [unwired: 1 in, 2 out]
            n189 = control-ref of="Position"() -> (w270:refnum<vi>)
            n190 = control-ref of="Position"() -> (w269:refnum<vi>)
            n191 = local read "Position"() -> (w271:dbl)
            n192 = local read "Position"() -> (w276:dbl)
            n193 = case shown="\"Left\", \"Right\"" w275 {
              tunnel: w269 -> [_ w280]
              tunnel: w270 -> [w279 _]
              tunnel: [w279 w280] -> w274
              frame "Down", "Up", Default {
              }
              frame "Left", "Right" {
              }
            }
            n194 = case shown="\"Up\"" w275 {
              tunnel: w271 -> [w282 _ _ w292]
              tunnel: "stepSize" -> [w283 w285 w288 w291]
              tunnel: [w281 w284 w287 w290] -> w273
              tunnel: w276 -> [_ w286 w289 _]
              frame "Right" {
                n195 = Add(x=w283, y=w282) -> (x+y=w281:dbl)
              }
              frame "Up" {
                n196 = Subtract(x=w286, y=w285) -> (x-y=w284:dbl)
              }
              frame "Down", Default {
                n197 = Add(x=w289, y=w288) -> (x+y=w287:dbl)
              }
              frame "Left" {
                n198 = Subtract(x=w292, y=w291) -> (x-y=w290:dbl)
              }
            }
            n199 = property class="DigNum (strict)"(reference=w274, "Val(Sgnl)"=w273) -> ()  [unwired: 1 in, 2 out]
          }
          event Timeout {
            n200 = event-data() -> ()  [unwired: 1 in, 2 out]
          }
          event Menu Selection (User) {
            n201 = event-data() -> ("MenuRef"=w298:refnum<k9>, "ItemTag"=w300:string)  [unwired: 1 in, 3 out]
            n202 = control-ref of="Main Tap"() -> (w295:refnum<vi>)
            n203 = call "ChangeMainTap.vi"("error in"=w297, "ItemTag"=w300, "reference"=w295) -> ("error out"=w301:errorcluster, "Boolean"=w302:bool)
            n204 = case shown="Error" w301 {
              selector: w301 -> [w303 _]
              tunnel: w298 -> [_ w309]
              tunnel: [_ w311] -> w299
              tunnel: w300 -> [_ w310]
              tunnel: [w303 errorcluster {"status"=FALSE, "code"=0, "source"=""} ("error IO")] -> w296
              frame No Error {
              }
              frame Error {
                n205 = local read "All Devices (h)"() -> (w304:string[])
                n206 = call "disableMenueItem.vi"("ItemTag"=w310, "All Devices (h)"=w304, "MenuRef"=w309) -> ("this is a Device(tag)"=w308:bool, "menu reference out"=w307:refnum<k9>)  [unwired: 1 in, 1 out]
                n207 = Get Menu Item Info(7:w310, 11:w309) -> (2:w313:string, 4:w314:bool)  [unwired: 1 in, 5 out]
                n208 = Not(x=w314) -> (.not. x?=w312:bool)
                n209 = case shown="Default" w310 {
                  selector: w310 -> [_ w320 _ _ _ _]
                  tunnel: w312 -> [w315 w318 w330 _ _ _]
                  tunnel: [_ _ TRUE _ _ _] -> w311
                  tunnel: w308 -> [_ w321 _ _ _ _]
                  tunnel: [w315 w319 w330 _ _ _] -> w306
                  frame "fixsize" {
                    n210 = control-ref of="This VI"() -> (w317:refnum<vi>)
                    n211 = Not(x=w315) -> (.not. x?=w316:bool)
                    n212 = property class="VI"(reference=w317, "Front Panel.Resizeable"=w316) -> ()  [unwired: 1 in, 2 out]
                    "fixsize" <- w315
                  }
                  frame Default {
                    n213 = case shown="True" w321 {
                      tunnel: w320 -> [_ w329]
                      tunnel: [_ w325] -> w319
                      tunnel: w318 -> [_ w325]
                      frame False {
                      }
                      frame True {
                        n214 = control-ref of="reset"() -> (w327:refnum<vi>)
                        n215 = control-ref of="This VI"() -> (w328:refnum<vi>)
                        n216 = call "getPortAndIP.vi"("Device Name"=w329, "This Vi"=w328) -> ("Remote Host"=w324:string, "port or service name"=w323:u16)  [unwired: 2 in, 3 out]
                        n217 = local write "port or service name"(w323) -> ()
                        n218 = local write "Remote Host"(w324) -> ()
                        n219 = property class="Bool (strict)"(reference=w327, "Val(Sgnl)"=TRUE ("Value (Signaling)")) -> ()  [unwired: 1 in, 2 out]
                        n220 = call "ConnectionFGV.vi"("command"=enum16{"get", "set", "init"}."set", "Remote Host in"=w324, "port or service name in"=w323) -> ()  [unwired: 7 in, 2 out]
                      }
                    }
                  }
                  frame "ratio" {
                    "ratio(h)" <- w330
                  }
                  frame "Local Saving Path" {
                    n221 = control-ref of="Local Saving Path"() -> (w332:refnum<vi>)
                    n222 = property class="Path"(reference=w332) -> (reference out=w335:refnum<vi>, "Value"=w336:path)  [unwired: 1 in, 1 out]
                    n223 = call "changePath.vi"("Local Saving in (h)"=w336) -> ("change (h)"=w334:bool, "Local Saving out (h)"=w333:path)  [unwired: 9 in]
                    n224 = case shown="True" w334 {
                      tunnel: w335 -> [_ w338]
                      tunnel: w333 -> [_ w337]
                      frame False {
                      }
                      frame True {
                        n225 = property class="Path"(reference=w338, "Val(Sgnl)"=w337) -> ()  [unwired: 1 in, 2 out]
                      }
                    }
                  }
                  frame "reset" {
                    n226 = control-ref of="reset"() -> (w340:refnum<vi>)
                    n227 = property class="Bool (strict)"(reference=w340, "Val(Sgnl)"=TRUE ("Value (Signaling)")) -> ()  [unwired: 1 in, 2 out]
                  }
                  frame "clear" {
                    n228 = control-ref of="reset"() -> (w342:refnum<vi>)
                    n229 = property class="Bool (strict)"(reference=w342, "Val(Sgnl)"=TRUE ("Value (Signaling)")) -> ()  [unwired: 1 in, 2 out]
                  }
                }
                n230 = Set Menu Item Info(6:w306, 7:w310, 10:w313, 11:w307) -> ()  [unwired: 3 in, 2 out]
              }
            }
          }
        }
        n231 = call "updateInicatorsMainVi.vi"("Data String out"=w165, "Boolean"=w166, "Array"=w167) -> ()  [unwired: 6 in, 3 out]
        n232 = call "updateInicatorsMainVi.vi"("Data String out"=w165, "Boolean"=w166, "Array"=w184, "Channel Selector"=w182, "error in"=w200) -> ("Data String out 2"=w191:string, "error out"=w187:errorcluster)  [unwired: 4 in, 1 out]
        n233 = control-ref of="Status"() -> (w180:refnum<vi>)
        n234 = control-ref of="Status"() -> (w179:refnum<vi>)
        n235 = control-ref of="all pos array"() -> (w175:refnum<vi>)
        n236 = call "stop.vi"("Boolean"=w194) -> ()
        n237 = call "StatusDataConnectionFGV.vi"("Command"=enum16{"get", "set", "init"}."get") -> ("Data Connection out"=→"Data Connection out":bool)  [unwired: 10 in]
        n238 = call "updateInicatorsMainVi.vi"("Data String out"=w165, "Boolean"=w166, "Array"=w183, "Channel Selector"=w181, "error in"=w187) -> ("error out"=w186:errorcluster)  [unwired: 4 in, 2 out]
        "error out" <- w186
        n239 = control-ref of="error (h)"() -> (w189:refnum<vi>)
        n240 = control-ref of="error message"() -> (w190:refnum<vi>)
        n241 = call "changeColorStatus.vi"("Enum in"=w179) -> ()  [unwired: 11 in]
        n242 = call "changeColorStatus.vi"("Enum in"=w180) -> ()  [unwired: 11 in]
        n243 = control-ref of="Main Tap"() -> (w169:refnum<vi>)
        n244 = control-ref of="all status array"() -> (w176:refnum<vi>)
        n245 = call "error.vi"("Boolean"=w166, "millisecond timer value"=w196, "reference"=w189, "error message"=w190) -> ("millisecond timer value 2"=w197:u32)
        n246 = call "allStatus.vi"("all pos array 2"=w175, "generic class reference"=w169, "Array in"=w176) -> ()  [unwired: 9 in]
      }
      n247 = local read "connections (hidden)"() -> (w162:variant[])
      n248 = call "Close UDP AND TCP connections.vi"("error in"=w163, "appended array"=w162) -> ()  [unwired: 6 in]
      "String" <- w153
    }
    frame #3 {
      n249 = control-ref of="Main  Control"() -> (w344:refnum<vi>)
      n250 = property class="TabCtl (strict)"(reference=w344, "Tabs Visible?"=TRUE) -> ()  [unwired: 1 in, 2 out]
      n251 = property class="TabCtl (strict)"(reference=w344, "Tab Location"=enum32{"Top", "Bottom", "Left", "Right"}."Bottom") -> ()  [unwired: 1 in, 2 out]
      n252 = flat-sequence {
        frame #0 {
          n253 = Wait (ms)(milliseconds to wait=u32 0) -> ()  [unwired: 1 out]
        }
        frame #1 {
        }
        frame #2 {
          n254 = control-ref of="This VI"() -> (w349:refnum<vi>)
          n255 = case shown="True" FALSE {
            tunnel: w349 -> [w350 w353]
            tunnel: [w350 w351] -> w348
            frame False {
            }
            frame True {
              n256 = property class="VI" props=["Front Panel.Open"](reference=w353) -> (reference out=w352:refnum<vi>)  [unwired: 1 in, 2 out]
              n257 = invoke class="VI" method="FP.Close"(reference=w352) -> (reference out=w351:refnum<vi>)  [unwired: 2 in, 2 out]
            }
          }
          n258 = Close Reference(reference=w348) -> ()  [unwired: 1 in, 1 out]
        }
      }
    }
  }
